vi "isFull.vi"(8 "error in (no error)":errorcluster, 9 "Capacity":i32, 11 "Object In":refnum<vi>) -> (0 "error out":errorcluster, 1 "Full?":bool, 3 "Mesh Ref":refnum<vi>)   [LabVIEW 2013, in "Trajectory Drawer.lvclass"]
uses:
  Trajectory Drawer.lvclass
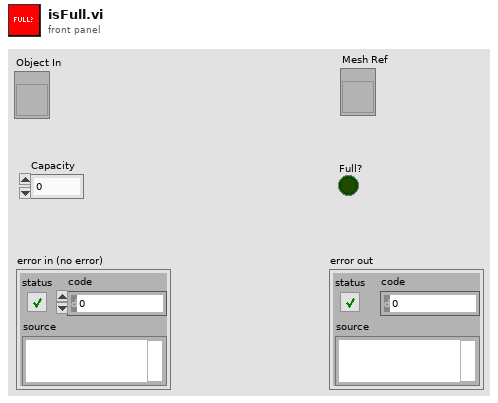
[diagram p1: front panel]
types:
  T1 = typedef "LV3DPointTypeDef.ctl" = cluster{"X":sgl, "Y":sgl, "Z":sgl}
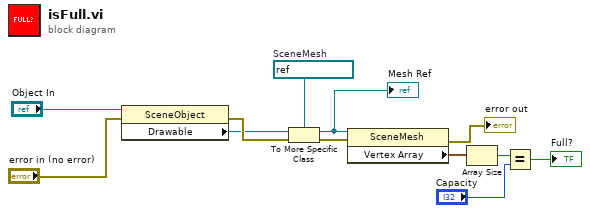
[diagram p0: block diagram]
diagram:
  w12 = refnum<vi> refnum  # SceneMesh
  n1 = property class="SceneObject"(reference="Object In", error in="error in (no error)") -> (error out=w9:errorcluster, "Drawable"=w8:refnum<vi>)  [unwired: 1 out]
  n2 = To More Specific Class(target class=w12, reference=w8, error in=w9) -> (specific class reference=w1:refnum<vi>, error out=w11:errorcluster)
  "Mesh Ref" <- w1
  n3 = property class="SceneMesh"(reference=w1, error in=w11) -> (error out=→"error out":errorcluster, "Vertex Array"=w7:T1[])  [unwired: 1 out]
  n4 = Array Size(array=w7) -> (size(s)=w3:i32)
  n5 = Equal?(x=w3, y="Capacity") -> (x = y?=→"Full?":bool)
